vi "String_match (SubVI).vi"(0 "channel id":string, 3 "input string":string, 5 "error in":errorcluster) -> (10 "match ?":i32, 14 "output string":string, 17 "match substring":string, 19 "error out":errorcluster)   [LabVIEW 2015]
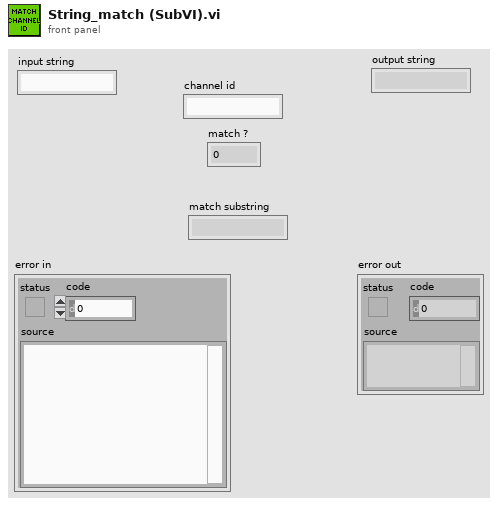
[diagram p1: front panel]
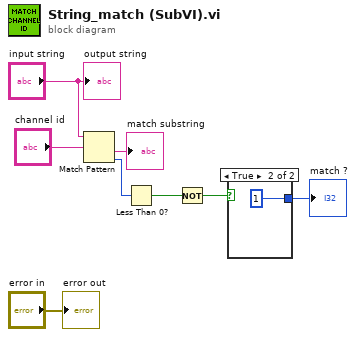
[diagram p0: block diagram]
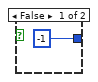
[diagram p2: hidden frame]
diagram:
  n1 = Match Pattern(string="input string", regular expression="channel id") -> (after substring=→"match substring":string, offset past match=w4:i32)  [unwired: 1 in, 2 out]
  n2 = Less Than 0?(x=w4) -> (x < 0?=w3:bool)
  n3 = Not(x=w3) -> (.not. x?=w2:bool)
  n4 = case shown="True" w2 {
    tunnel: [-1 ("match ?") 1 ("match ?")] -> w1
    frame False {
    }
    frame True {
    }
  }
  "match ?" <- w1
  "output string" <- "input string"
  "error out" <- "error in"
